vi "Serial Port Init.vi"(1 "flow control etc.":T1={"input XON/XOFF"=FALSE, "input HW Handshake"=FALSE, "input alt HW HShk"=FALSE, "output XON/XOFF"=FALSE, "output HW Handshake"=FALSE, "output alt HW HShk"=FALSE, "XOFF byte "=19, "XON byte"=17, "parity error byte"=0} {"parity error byte" format="%x"; "XON byte" format="%x"; "XOFF byte" format="%x"}, 2 "parity":T2(ring), 3 "buffer size":u16, 4 "stop bits":enum16{"1 bit", "1.5 bits", "2 bits"}(ring), 5 "data bits":u16=8 min=5 max=8 step=1, 6 "baud rate":u32=9600, 7 "port number":i32) -> (0 "error code":i32)   [LabVIEW 2013]
doc: "Initializes the selected serial port to the settings you specify."
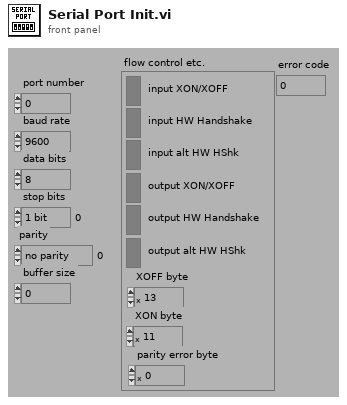
[diagram p1: front panel]
types:
  T1 = cluster{"input XON/XOFF":bool, "input HW Handshake":bool, "input alt HW HShk":bool, "output XON/XOFF":bool, "output HW Handshake":bool, "output alt HW HShk":bool, "XOFF byte ":u8, "XON byte":u8, "parity error byte":u16}
  T2 = enum16{"no parity", "odd parity", "even parity", "mark parity", "space parity"}
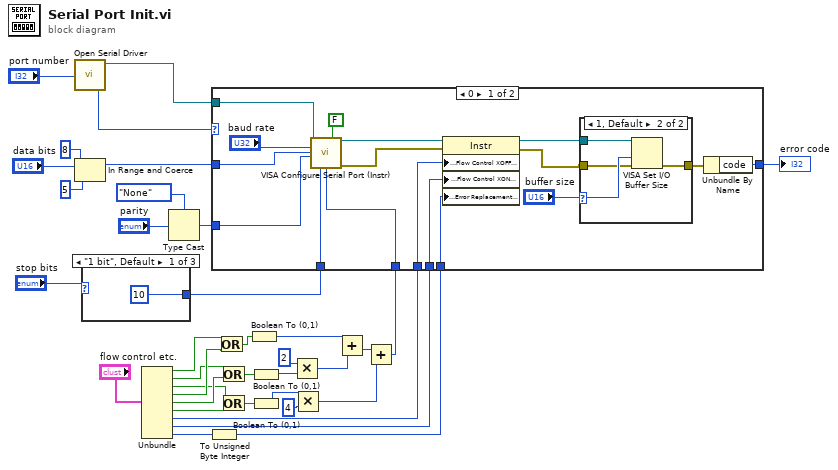
[diagram p0: block diagram]
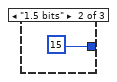
[diagram p2: hidden frame]
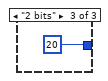
[diagram p3: hidden frame]
diagram:
  n1 = call "Open Serial Driver.vi"("port number"="port number") -> ("input refnum"=w31:refnum<visa-resource-name>, "output error"=w32:i32)  [unwired: 2 out]
  n2 = In Range and Coerce(upper limit=u16 8, x="data bits", lower limit=u16 5) -> (coerced(x)=w30:u16)  [unwired: 1 out]
  n3 = case shown="\"1 bit\", Default" "stop bits" {
    tunnel: [u16 10 u16 15 u16 20] -> w25
    frame "1 bit", Default {
    }
    frame "1.5 bits" {
    }
    frame "2 bits" {
    }
  }
  n4 = Unbundle("flow control etc.") -> ("input XON/XOFF"=w18:bool, "input HW Handshake"=w15:bool, "input alt HW HShk"=w13:bool, "output XON/XOFF"=w17:bool, "output HW Handshake"=w14:bool, "output alt HW HShk"=w12:bool, "XOFF byte"=w22:u8, "XON byte"=w21:u8, "parity error byte"=w20:u16)
  n5 = Type Cast(type=enum16{"None", "Odd", "Even", "Mark", "Space"}."None" ("parity (0:none)"), x="parity") -> (*(type *) &x=w27:enum16{"None", "Odd", "Even", "Mark", "Space"})
  n6 = To Unsigned Byte Integer(number=w20) -> (unsigned 8bit integer=w19:u8)
  n7 = Or(x=w18, y=w17) -> (x .or. y?=w16:bool)
  n8 = Or(x=w15, y=w14) -> (x .or. y?=w11:bool)
  n9 = Or(x=w13, y=w12) -> (x .or. y?=w10:bool)
  n10 = Boolean To (0,1)(Boolean=w16) -> (0, 1=w5:i16)
  n11 = Boolean To (0,1)(Boolean=w11) -> (0, 1=w8:i16)
  n12 = Boolean To (0,1)(Boolean=w10) -> (0, 1=w6:i16)
  n13 = Multiply(x=u16 2 ("y"), y=w8) -> (x*y=w4:u16)
  n14 = Multiply(x=w6, y=u16 4) -> (x*y=w3:u16)
  n15 = Add(x=w5, y=w4) -> (x+y=w2:u16)
  n16 = Add(x=w2, y=w3) -> (x+y=w1:u16)
  n17 = case shown="0" w32 {
    selector: w32 -> [_ w62]
    tunnel: w31 -> [w55 _]
    tunnel: w30 -> [w53 _]
    tunnel: w27 -> [w52 _]
    tunnel: w25 -> [w51 _]
    tunnel: [w48 w62] -> w24
    tunnel: w22 -> [w43 _]
    tunnel: w21 -> [w42 _]
    tunnel: w19 -> [w41 _]
    tunnel: w1 -> [w40 _]
    frame 0 {
      n18 = call "VISA Configure Serial Port (Instr).vi"("VISA resource name"=w55, "Enable Termination\nChar (T)"=FALSE ("Enable Termination\nChar (T)"), "baud rate (9600)"="baud rate", "data bits (8)"=w53, "parity (0:none)"=w52, "stop bits (10: 1 bit)"=w51, "flow control (0:none)"=w40) -> ("VISA resource name out"=w47:refnum<visa-resource-name>, "error out"=w45:errorcluster)  [unwired: 7 in]
      n19 = property class="Instr"(reference=w47, error in=w45, "Serial Settings:Flow Control XOFF Character"=w43, "Serial Settings:Flow Control XON Character"=w42, "Serial Settings:Error Replacement Character"=w41) -> (reference out=w46:refnum<visa-resource-name>, error out=w44:errorcluster)
      n20 = case shown="1, Default" "buffer size" {
        selector: "buffer size" -> [_ w60]
        tunnel: w46 -> [_ w61]
        tunnel: w44 -> [w57 w59]
        tunnel: [w57 w58] -> w49
        frame 0 {
        }
        frame 1, Default {
          n21 = VISA Set I/O Buffer Size(VISA resource name=w61, size (4096)=w60, error in (no error)=w59) -> (error out=w58:errorcluster)  [unwired: 1 in, 1 out]
        }
      }
      n22 = Unbundle By Name(w49) -> ("code"=w48:i32)
    }
    frame 1, Default {
    }
  }
  "error code" <- w24
